vi "RT Driver VI.vi"(7 "Operation":T1, 11 "Device Reference in":T2 format="%.0x") -> (0 "Error Code":i32)   [LabVIEW 2017, in "DSF Engine.lvlib"]
uses:
  DSF Engine.lvlib
  <vilib>/NI Veristand/Custom Device API/Custom Device Item Ref.ctl
  <vilib>/NI Veristand/Custom Device API/Hardware Interface Driver VI Operation.ctl
  VeriStand DSF/VeriStand DSF.lvclass
  State Data.ctl
  <vilib>/NI Veristand/Custom Device API/Global Data Refs.vi
  DSF Core.lvlibp/Classes/Framework/Increment Framework Cycle.vi
  DSF Core.lvlibp/Classes/Framework/Cycle Begin.vi
  DSF Core.lvlibp/Classes/Framework/Receive.vi
  <vilib>/NI Veristand/Custom Device API/Custom Device API.lvlib
  DSF Core.lvlibp/Classes/Framework/Framework.lvclass
  Shared/DSF Shared.lvlib
  DSF Core.lvlibp/Classes/Thread/Thread Options.ctl
  DSF Core.lvlibp/Classes/Thread/Thread.lvclass
  C:/Git/niveristand-data-sharing-framework-custom-device/VeriStand/Data Sharing Custom Device/Source/DSF Core.lvlibp/Classes/Framework/Framework.lvclass
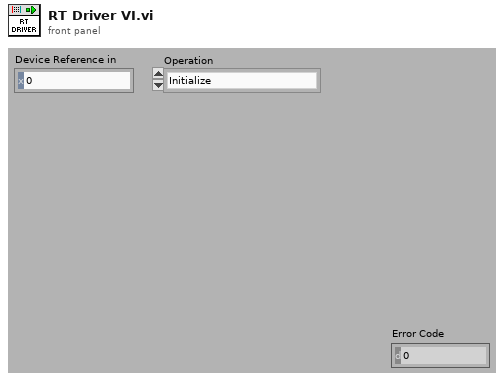
[diagram p1: front panel]
types:
  T1 = typedef "Custom Device API.lvlib/Hardware Interface Driver VI Operation.ctl" = enum16{"Initialize", "Start", "Read Data from HW", "Write Data to HW", "Close"}
  T2 = typedef "Custom Device API.lvlib/Custom Device Item Ref.ctl" = u64
  T3 = typedef "DSF Engine.lvlib/State Data.ctl" = cluster{"show error dialog":bool}
  T4 = typedef "DSF Core.lvlibp/Thread.lvclass/Thread Options.ctl" = cluster{"Show FP On Call":bool, "Close FP After Call":bool, "Allow Debugging":bool}
  T5 = typedef "DSF Core.lvlibp/Framework.lvclass/Framework Options.ctl" = cluster{"FIFO Options":T6, "Thread Options":T4, "Plugin Options":T7, "Performance Options":T8, "Data Server Options":T9}
  T6 = typedef "DSF Core.lvlibp/Framework.lvclass/DSF FIFO Options.ctl" = cluster{"Infinite Timeouts":bool}
  T7 = typedef "DSF Core.lvlibp/Framework.lvclass/DSF Plugin Options.ctl" = cluster{"Default Components":bool}
  T8 = typedef "DSF Core.lvlibp/DSF Performance Options.ctl" = cluster{"Measure Period":bool, "Measure Rx/Tx Duration":bool}
  T9 = typedef "DSF Core.lvlibp/Framework.lvclass/Data Server Options.ctl" = cluster{"Enable Data Server":bool, "Period":u32}
  T10 = typedef "Custom Device API.lvlib/Data Table Ref.ctl" = cluster{"Ptr.Beg":u64, "Ptr.End":u64}
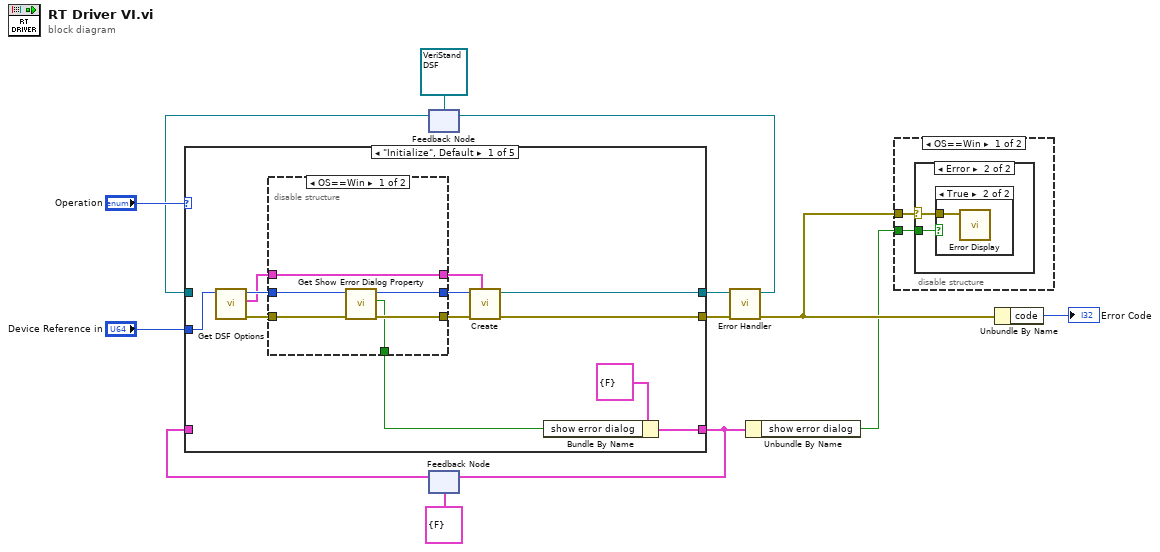
[diagram p0: block diagram]
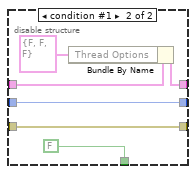
[diagram p2: hidden frame]
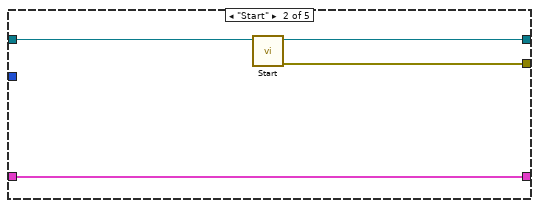
[diagram p3: hidden frame]
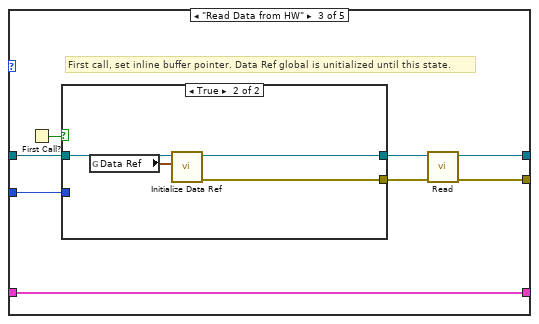
[diagram p4: hidden frame]
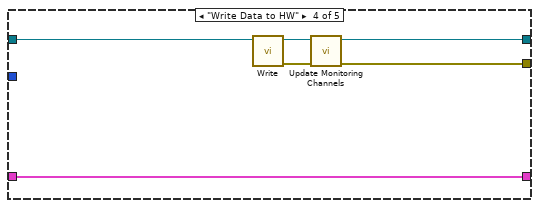
[diagram p6: hidden frame]
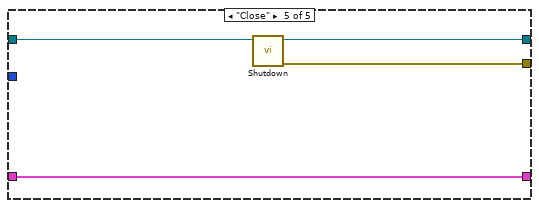
[diagram p7: hidden frame]
diagram:
  n1 = feedback #1(refnum<class "VeriStand DSF.lvclass"> refnum ("Data Sharing Framework Engine.lvlib:VeriStand Data Sharing Framework.lvclass")) -> (w10:refnum<class "VeriStand DSF.lvclass">)
  n2 = feedback #2(T3 {"show error dialog"=FALSE} ("state data")) -> (w8:T3)
  n3 = case shown="\"Initialize\", Default" "Operation" {
    tunnel: [w25 w40 w47 w56 w62] -> w6
    tunnel: w10 -> [_ w41 w48 w60 w64]
    tunnel: "Device Reference in" -> [w24 _ w43 _ _]
    tunnel: [w14 w39 w44 w55 w63] -> w7
    tunnel: [w21 w38 w42 w59 w61] -> w3
    tunnel: w8 -> [_ w38 w42 w59 w61]
    frame "Initialize", Default {
      n4 = call "Get DSF Options.vi"("Item Ref in"=w24) -> ("error out"=w20:errorcluster, "options"=w15:T5, "Item Ref out"=w19:T2)  [unwired: 8 in]
      n5 = disable-structure shown="OS==Win" {
        disable-tunnel: [w30 w35] -> w23
        disable-tunnel: w15 -> [w30 w36]
        disable-tunnel: w20 -> [w26 w33]
        disable-tunnel: w19 -> [w27 w34]
        disable-tunnel: [w31 w34] -> w18
        disable-tunnel: [w29 w33] -> w17
        disable-tunnel: [w28 FALSE ("launch data viewer")] -> w16
        frame condition #0 (active) {
          n6 = call "Get Show Error Dialog Property.vi"("error in (no error)"=w26, "Item Ref in"=w27) -> ("error out"=w29:errorcluster, "show error dialog"=w28:bool, "Item Ref out"=w31:T2)  [unwired: 7 in]
        }
        frame condition #1 {
          n7 = Bundle By Name(cluster=w36, "Thread Options"=T4 {"Show FP On Call"=FALSE, "Close FP After Call"=FALSE, "Allow Debugging"=FALSE}) -> (w35:T5)
        }
      }
      n8 = call "Create.vi"("options"=w23, "error in (no error)"=w17, "Device Item Ref"=w18) -> ("error out"=w14:errorcluster, "VeriStand Framework"=w25:refnum<class "VeriStand DSF.lvclass">)  [unwired: 7 in]
      n9 = Bundle By Name(cluster=T3 {"show error dialog"=FALSE} ("state data"), "show error dialog"=w16) -> (w21:T3)
    }
    frame "Start" {
      n10 = call-dynamic "Start.vi"("VeriStand Data Sharing Framework in"=w41) -> ("error out"=w39:errorcluster, "VeriStand Data Sharing Framework out"=w40:refnum<class "VeriStand DSF.lvclass">)  [unwired: 9 in]
    }
    frame "Read Data from HW" {
      # "First call, set inline buffer pointer. Data Ref global is unitialized until this state."
      n11 = First Call?() -> (First Call?: T/F=w49:bool)
      n12 = case shown="True" w49 {
        tunnel: w48 -> [w50 w54]
        tunnel: [w50 w52] -> w46
        tunnel: [_ w51] -> w45
        tunnel: w43 -> [_ _]
        frame False {
        }
        frame True {
          n13 = global read "Global Data Refs.vi" "Data Ref"() -> (w53:T10)
          n14 = call "Initialize Data Ref.vi"("Data Ref"=w53, "VeriStand DSF in"=w54) -> ("error out"=w51:errorcluster, "VeriStand DSF out"=w52:refnum<class "VeriStand DSF.lvclass">)  [unwired: 8 in]
        }
      }
      n15 = call "Read.vi"("error in (no error)"=w45, "VeriStand DSF in"=w46) -> ("error out"=w44:errorcluster, "VeriStand DSF out"=w47:refnum<class "VeriStand DSF.lvclass">)  [unwired: 8 in]
    }
    frame "Write Data to HW" {
      n16 = call "Write.vi"("VeriStand DSF in"=w60) -> ("error out"=w57:errorcluster, "VeriStand DSF out"=w58:refnum<class "VeriStand DSF.lvclass">)  [unwired: 9 in]
      n17 = call "Update Monitoring Channels.vi"("error in (no error)"=w57, "VeriStand DSF in"=w58) -> ("error out"=w55:errorcluster, "VeriStand DSF out"=w56:refnum<class "VeriStand DSF.lvclass">)  [unwired: 8 in]
    }
    frame "Close" {
      n18 = call-dynamic "Shutdown.vi"("VeriStand Data Sharing Framework in"=w64) -> ("error out"=w63:errorcluster, "VeriStand Data Sharing Framework out"=w62:refnum<class "VeriStand DSF.lvclass">)  [unwired: 9 in]
    }
  }
  n19 = feedback-in #2(w3) -> ()
  n20 = call "Error Handler.vi"("error in (no error)"=w7, "Framework in"=w6) -> ("error out"=w5:errorcluster, "Framework out"=w1:refnum<class "VeriStand DSF.lvclass">)  [unwired: 8 in]
  n21 = feedback-in #1(w1) -> ()
  n22 = Unbundle By Name(w3) -> ("show error dialog"=w2:bool)
  n23 = disable-structure shown="OS==Win" {
    disable-tunnel: w5 -> [w66 _]
    disable-tunnel: w2 -> [w65 _]
    frame condition #0 (active) {
      n24 = case shown="Error" w66 {
        selector: w66 -> [_ w68]
        tunnel: w65 -> [_ w67]
        frame No Error {
        }
        frame Error {
          n25 = case shown="True" w67 {
            tunnel: w68 -> [_ w69]
            frame False {
            }
            frame True {
              n26 = call "Error Display.vi"("error"=w69) -> ()  [unwired: 11 in]
            }
          }
        }
      }
    }
    frame condition #1 {
    }
  }
  n27 = Unbundle By Name(w5) -> ("code"=→"Error Code":i32)
